vi "IntegraMeter_ContinuousReader.vi"() -> ()   [LabVIEW 2024]
panel:
  out "number of measurements":i32
  out "Laser Energy (J)":dbl
  in  "stop":bool
  in  "VISA resource name":refnum<visa-resource-name>
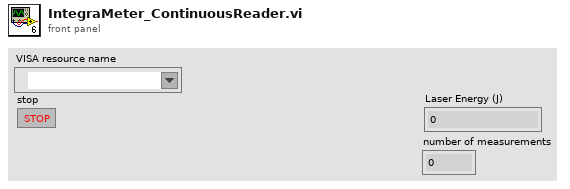
[diagram p1: front panel]
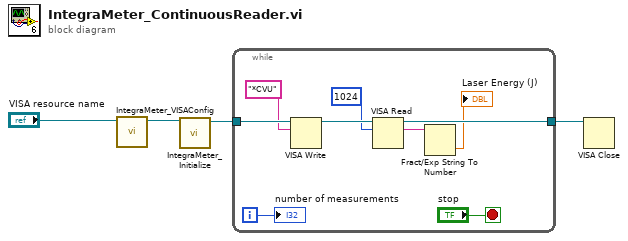
[diagram p0: block diagram]
diagram:
  n1 = call "IntegraMeter_VISAConfig.vi"("VISA resource name"="VISA resource name") -> ("reference out"=w4:refnum<visa-resource-name>)  [unwired: 9 in, 1 out]
  n2 = call "IntegraMeter_Initialize.vi"("VISA resource name"=w4) -> ("VISA resource name out"=w2:refnum<visa-resource-name>)  [unwired: 9 in, 1 out]
  n3 = while {
    tunnel: w2 -> [w13]
    tunnel: [w11] -> w1
    i -> [w5]
    stop <- "stop" stop-if-true
    n4 = VISA Write(VISA resource name=w13, write buffer="*CVU") -> (VISA resource name out=w12:refnum<visa-resource-name>)  [unwired: 1 in, 2 out]
    n5 = VISA Read(VISA resource name=w12, byte count=u32 1024) -> (VISA resource name out=w11:refnum<visa-resource-name>, read buffer=w7:string)  [unwired: 1 in, 2 out]
    n6 = Fract/Exp String To Number(string=w7) -> (number=→"Laser Energy (J)":dbl)  [unwired: 3 in, 1 out]
    "number of measurements" <- w5
  }
  n7 = VISA Close(VISA resource name=w1) -> ()  [unwired: 1 in, 1 out]
